vi "Test Find Callers - NEEDS CLEANUP.vi"   [LabVIEW 2020]
uses:
  source/JKI SM/JKI SM.lvclass
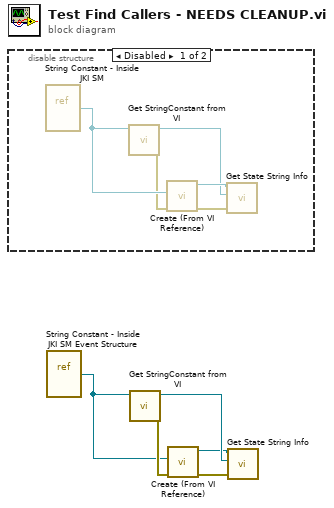
[diagram p0: block diagram]
diagram:
  n1 = disable-structure shown="Disabled" {
    frame Disabled {
      n2 = vi-ref "String Constant - Inside JKI SM.vi"() -> (w10:refnum<vi>)
      n3 = call "Get StringConstant from VI.vi"("VI in"=w10) -> ("error out"=w7:errorcluster, "StringConstant out"=w8:refnum<vi>)  [unwired: 9 in]
      n4 = call "Create (From VI Reference).vi"("error in (no error)"=w7, "VI"=w10) -> ("error out"=w6:errorcluster, "JKI SM out"=w9:refnum<class "JKI SM.lvclass">)  [unwired: 8 in]
      n5 = call "Get State String Info.vi"("error in (no error)"=w6, "GObj Refnum in"=w8, "JKI SM in"=w9) -> ()  [unwired: 5 in, 4 out]
    }
    frame Enabled {
    }
  }
  n6 = vi-ref "String Constant - Inside JKI SM Event Structure.vi"() -> (w1:refnum<vi>)
  n7 = call "Get StringConstant from VI.vi"("VI in"=w1) -> ("error out"=w4:errorcluster, "StringConstant out"=w3:refnum<vi>)  [unwired: 9 in]
  n8 = call "Create (From VI Reference).vi"("error in (no error)"=w4, "VI"=w1) -> ("error out"=w5:errorcluster, "JKI SM out"=w2:refnum<class "JKI SM.lvclass">)  [unwired: 8 in]
  n9 = call "Get State String Info.vi"("error in (no error)"=w5, "GObj Refnum in"=w3, "JKI SM in"=w2) -> ()  [unwired: 5 in, 4 out]
